vi "create table mesages.vi"(10 "serial_n name":string="serial_n1_seq", 11 "table name":string="FA") -> (3 "create table parameters":string)   [LabVIEW 2019, in "PostgreSQL.lvlib"]
uses:
  PostgreSQL.lvlib
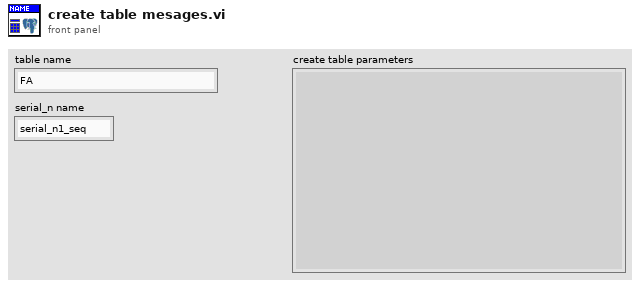
[diagram p1: front panel]
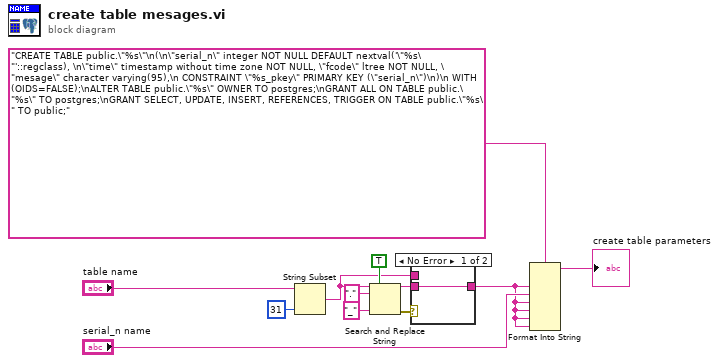
[diagram p0: block diagram]
diagram:
  n1 = String Subset(string="table name", length (rest)=31 ("offset (0)")) -> (substring=w7:string)  [unwired: 1 in]
  n2 = Search and Replace String(replace all?=TRUE ("replace all? (F)"), input string=w7, search string=".", replace string="_" ("replace string (\"\")")) -> (result string=w9:string, error out=w10:errorcluster)  [unwired: 4 in, 2 out]
  n3 = case shown="No Error" w10 {
    tunnel: w9 -> [w13 _]
    tunnel: [w13 w14] -> w3
    tunnel: w7 -> [_ w14]
    frame No Error {
    }
    frame Error {
    }
  }
  n4 = Format Into String(format string="CREATE TABLE public.\"%s\"\n(\n\"serial_n\" integer NOT NULL DEFAULT nextval('\"%s\"'::regclass), \n\"time\" timestamp without time zone NOT NULL, \"fcode\" ltree NOT NULL, \"mesage\" character varying(95),\n CONSTRAINT \"%s_pkey\" PRIMARY KEY (\"serial_n\")\n)\n WITH (OIDS=FALSE);\nALTER TABLE public.\"%s\" OWNER TO postgres;\nGRANT ALL ON TABLE public.\"%s\" TO postgres;\nGRANT SELECT, UPDATE, INSERT, REFERENCES, TRIGGER ON TABLE public.\"%s\" TO public;", w3, "serial_n name", w3, w3, w3, w3) -> (resulting string=→"create table parameters":string)  [unwired: 2 in, 1 out]
